vi "Handle Exception.vi"(7 "Processing In":refnum<class "Processing.lvclass">, 8 "error in (no error)":errorcluster, 11 "Error Logger in":refnum<class "Error Logger.lvclass">) -> (0 "error out":errorcluster, 5 "Processing":refnum<class "Processing.lvclass">)   [LabVIEW 2020, in "Summer of LabVIEW.lvlib" / "Error Logger.lvclass"]
uses:
  Error Logger.lvclass
  Error Logger.lvclass/Error Logger.ctl
  SOL-Server/SOL-Server.lvclass
  <vilib>/IlluminatedG/IG HTTP Server/HTTP Server/Processing/Processing.lvclass
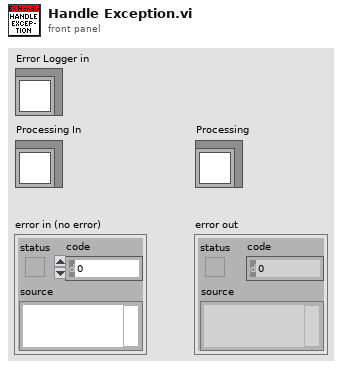
[diagram p1: front panel]
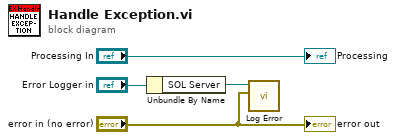
[diagram p0: block diagram]
diagram:
  n1 = Unbundle By Name("Error Logger in") -> ("SOL Server"=w3:refnum<class "SOL-Server.lvclass">)
  n2 = call "Log Error.vi"("error in (no error)"="error in (no error)", "SOL-Server in"=w3) -> ()  [unwired: 9 in, 1 out]
  "error out" <- "error in (no error)"
  "Processing" <- "Processing In"
